vi "Pokayoka signal.vi"() -> (1 "IL Sensor":T1, 2 "output cluster":T2)   [LabVIEW 2015]
uses:
  Galobal variable_TI.vi
panel:
  # "1 emergency\n4 pressure\n5  &6 saftey\n27 slide servo Home RS\n28 Servo Fault\n33LVDT UP RS\n31 Pressing UP RS \n 38 Deg dw rs"
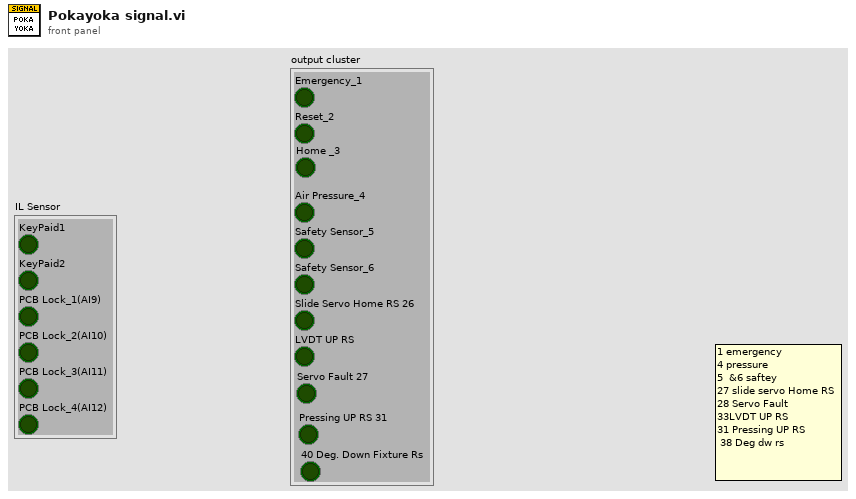
[diagram p1: front panel]
types:
  T1 = cluster{"KeyPaid1":bool, "KeyPaid2":bool, "PCB Lock_1(AI9)":bool, "PCB Lock_2(AI10)":bool, "PCB Lock_3(AI11)":bool, "PCB Lock_4(AI12)":bool}
  T2 = cluster{"Emergency_1":bool, "Reset_2":bool, "Home _3":bool, "Air Pressure_4":bool, "Safety Sensor_5":bool, "Safety Sensor_6":bool, "Slide Servo Home RS 26":bool, "LVDT UP RS":bool, "Servo Fault 27":bool, "Pressing UP RS 31":bool, "40 Deg. Down Fixture Rs":bool}
  T3 = cluster{"Emergency_1":bool, "Reset_2":bool, "Home _3":bool, "Air Pressure_4":bool, "Safety Sensor_5":bool, "Safety Sensor_6":bool, "Slide Servo Home RS 27":bool, "LVDT UP RS":bool, "Servo Fault 28":bool, "Pressing UP RS 31":bool, "40 Deg. Down Fixture Rs":bool}
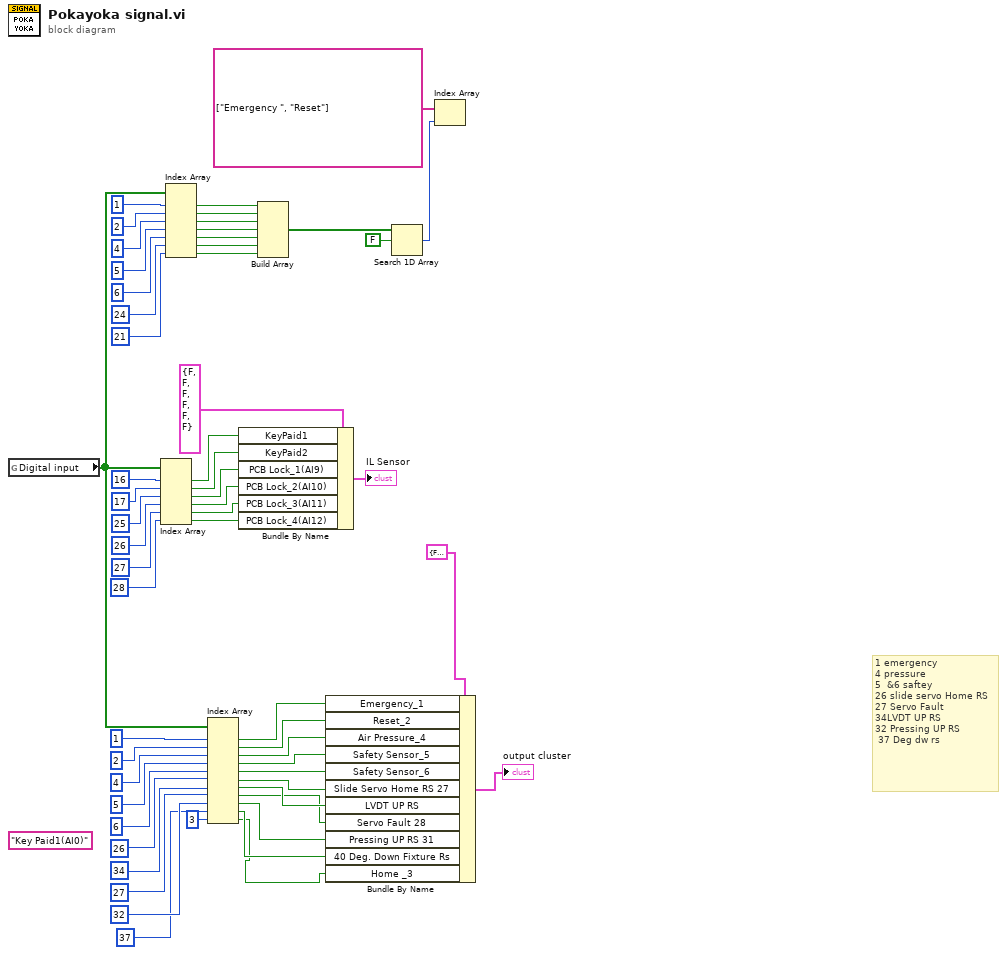
[diagram p0: block diagram]
diagram:
  (unwired) "Key Paid1(AI0)"
  # "1 emergency\n4 pressure\n5  &6 saftey\n26 slide servo Home RS\n27 Servo Fault\n34LVDT UP RS\n32 Pressing UP RS \n 37 Deg dw rs"
  n1 = global read "Galobal variable_TI.vi" "Digital input"() -> (w18:bool[])
  n2 = Index Array(array=w18, index #1=16 ("index"), index #2=17 ("index"), index #3=25 ("index"), index #4=26 ("index"), index #5=27 ("index"), index #6=28 ("index")) -> (element #1=w16:bool, element #2=w15:bool, element #3=w14:bool, element #4=w13:bool, element #5=w12:bool, element #6=w11:bool)
  n3 = Index Array(array=w18, index #1=1 ("index"), index #2=2 ("index"), index #3=4 ("index"), index #4=5 ("index"), index #5=6 ("index"), index #6=24 ("index"), index #7=21 ("index")) -> (element #1=w35:bool, element #2=w34:bool, element #3=w33:bool, element #4=w32:bool, element #5=w31:bool, element #6=w30:bool, element #7=w29:bool)
  n4 = Index Array(array=w18, index #1=1 ("index"), index #2=2 ("index"), index #3=4 ("index"), index #4=5 ("index"), index #5=6 ("index"), index #6=26 ("index"), index #7=34 ("index"), index #8=27 ("index"), index #9=32 ("index"), index #10=37 ("index"), index #11=3 ("index")) -> (element #1=w57:bool, element #2=w56:bool, element #3=w55:bool, element #4=w54:bool, element #5=w53:bool, element #6=w52:bool, element #7=w51:bool, element #8=w8:bool, element #9=w7:bool, element #10=w4:bool, element #11=w1:bool)
  n5 = Bundle By Name(cluster=T1 {"KeyPaid1"=FALSE, "KeyPaid2"=FALSE, "PCB Lock_1(AI9)"=FALSE, "PCB Lock_2(AI10)"=FALSE, "PCB Lock_3(AI11)"=FALSE, "PCB Lock_4(AI12)"=FALSE} ("PCB LOCK"), "KeyPaid1"=w16, "KeyPaid2"=w15, "PCB Lock_1(AI9)"=w14, "PCB Lock_2(AI10)"=w13, "PCB Lock_3(AI11)"=w12, "PCB Lock_4(AI12)"=w11) -> (→"IL Sensor":T1)
  n6 = Build Array(w35, w34, w33, w32, w31, w30, w29) -> (w28:bool[])
  n7 = Bundle By Name(cluster=T3 {"Emergency_1"=FALSE, "Reset_2"=FALSE, "Home _3"=FALSE, "Air Pressure_4"=FALSE, "Safety Sensor_5"=FALSE, "Safety Sensor_6"=FALSE, "Slide Servo Home RS 27"=FALSE, "LVDT UP RS"=FALSE, "Servo Fault 28"=FALSE, "Pressing UP RS 31"=FALSE, "40 Deg. Down Fixture Rs"=FALSE} ("output cluster 2"), "Emergency_1"=w57, "Reset_2"=w56, "Air Pressure_4"=w55, "Safety Sensor_5"=w54, "Safety Sensor_6"=w53, "Slide Servo Home RS 27"=w52, "LVDT UP RS"=w51, "Servo Fault 28"=w8, "Pressing UP RS 31"=w7, "40 Deg. Down Fixture Rs"=w4, "Home _3"=w1) -> (→"output cluster":T3)
  n8 = Search 1D Array(1D array=w28, element=FALSE) -> (index of element=w26:i32)  [unwired: 1 in]
  n9 = Index Array(array=string[] ["Emergency ", "Reset"], index=w26) -> ()  [unwired: 1 out]
